vi "Send Power To Forward Drive.vi"(8 "error in (no error)":errorcluster, 9 "Right Power":dbl min=-1.0 max=1.0, 10 "Left Power":dbl min=-1.0 max=1.0, 11 "Logical Driver in":refnum<class "Driver.lvclass">) -> (0 "error out":errorcluster, 3 "Logical Driver out":refnum<class "Driver.lvclass">)   [LabVIEW 2014, in "Driver.lvlib" / "Driver.lvclass"]
uses:
  Driver.lvclass
  Forward Drive/Forward Drive Commands/Drive by Power/Drive by Power.lvclass
  Robot Actor Framework/Command Processor Actor/Command Processor Actor Messages/Start Command/Start Command Msg.lvclass/Start Command Msg.ctl
  <vilib>/ActorFramework/Message Enqueuer/Message Enqueuer.lvclass/Message Enqueuer.ctl
  <vilib>/ActorFramework/Message Enqueuer/Enqueue.vi
  <vilib>/ActorFramework/Message Priority Queue/Priority Enqueue.vi
  Robot Actor Framework/Command Processor Actor/Command Processor Actor Messages/Start Command/Start Command Msg.lvclass
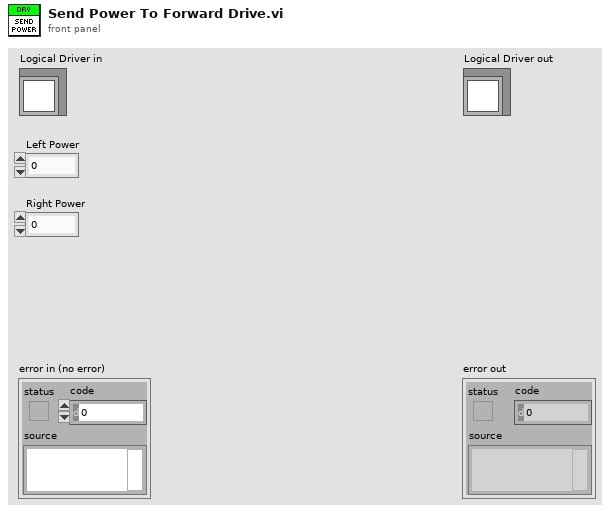
[diagram p1: front panel]
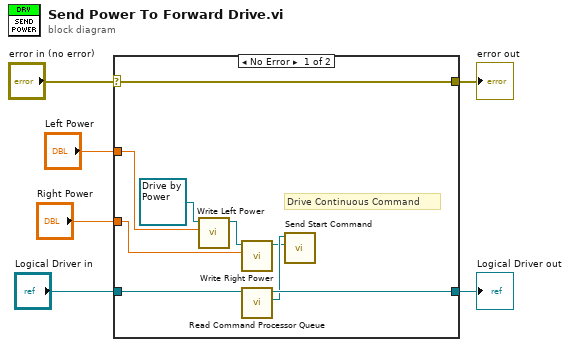
[diagram p0: block diagram]
diagram:
  n1 = case shown="No Error" "error in (no error)" {
    selector: "error in (no error)" -> [w15 w17]
    tunnel: [w15 w17] -> w5
    tunnel: [w13 w16] -> w3
    tunnel: "Logical Driver in" -> [w14 w16]
    tunnel: "Left Power" -> [w8 _]
    tunnel: "Right Power" -> [w7 _]
    frame No Error {
      # "Drive Continuous Command"
      n2 = call-dynamic "Write Left Power.vi"("Left Power"=w8, "Drive Continuous Cmd in"=refnum<class "Drive by Power.lvclass"> refnum ("Logical Forward Drive.lvlib:Drive Continuous Cmd.lvclass")) -> ("Drive Continuous Cmd out"=w10:refnum<class "Drive by Power.lvclass">)  [unwired: 8 in, 1 out]
      n3 = call-dynamic "Write Right Power.vi"("Right Power"=w7, "Drive Continuous Cmd in"=w10) -> ("Drive Continuous Cmd out"=w9:refnum<class "Drive by Power.lvclass">)  [unwired: 8 in, 1 out]
      n4 = call-dynamic "Read Command Processor Queue.vi"("System Actor in"=w14) -> ("Actor Framework:Message Enqueuer"=w12:refnum<class "Message Enqueuer.lvclass">, "System Actor out"=w13:refnum<class "Driver.lvclass">)  [unwired: 7 in, 2 out]
      n5 = call "Send Start Command.vi"("Robot Actors.lvlib:Command.lvlib:Command.lvclass"=w9, "Message Enqueuer"=w12) -> ()  [unwired: 8 in, 2 out]
    }
    frame Error {
    }
  }
  "error out" <- w5
  "Logical Driver out" <- w3
